vi "Configuracion_ADS_operar.vi"(7 "Direccion":i16, 9 "Configuracion ADS1263":T1 {"Muestras" items=["50", "250", "1000", "2000", "5000", "10000", "15000", "30000"]; "PGA" items=["1", "2", "4", "8", "16", "32"]; "Muestreo" items=["2.5 SPS", "5 SPS", "10 SPS", "16.6 SPS", "20 SPS", "50 SPS", "60 SPS", "100 SPS", "400 SPS", "1200 SPS", "2400 SPS", "4800 SPS", "7200 SPS", "14400 SPS", "19200 SPS", "38400 SPS"]}, 10 "ENVIAR_CONFI":bool) -> (1 "Muestras":i32, 2 "Configuracion":string)   [LabVIEW 2022 SP3]
panel:
  # "Velocidad de muestreo"
  # "PGA del sistema"
  # "HABILITAR MODO DIFERENCIAL 1 Y 2"
  # "HABILITAR MODO DIFERENCIAL 3 Y 4"
  # "FILTRO PARA AC1 Y AC2"
  # "100Hz"
  # "500Hz"
  # "FILTRO PARA AC3 Y AC4"
  # "100Hz"
  # "500Hz"
  # "MODO DE OPERACION DEMANDA"
  # "MODO DE OPERACION CONTROLADA"
  # "Cantidad de muestras tomadas"
  # "Recibir por LoRa"
  # "Recibir por SD"
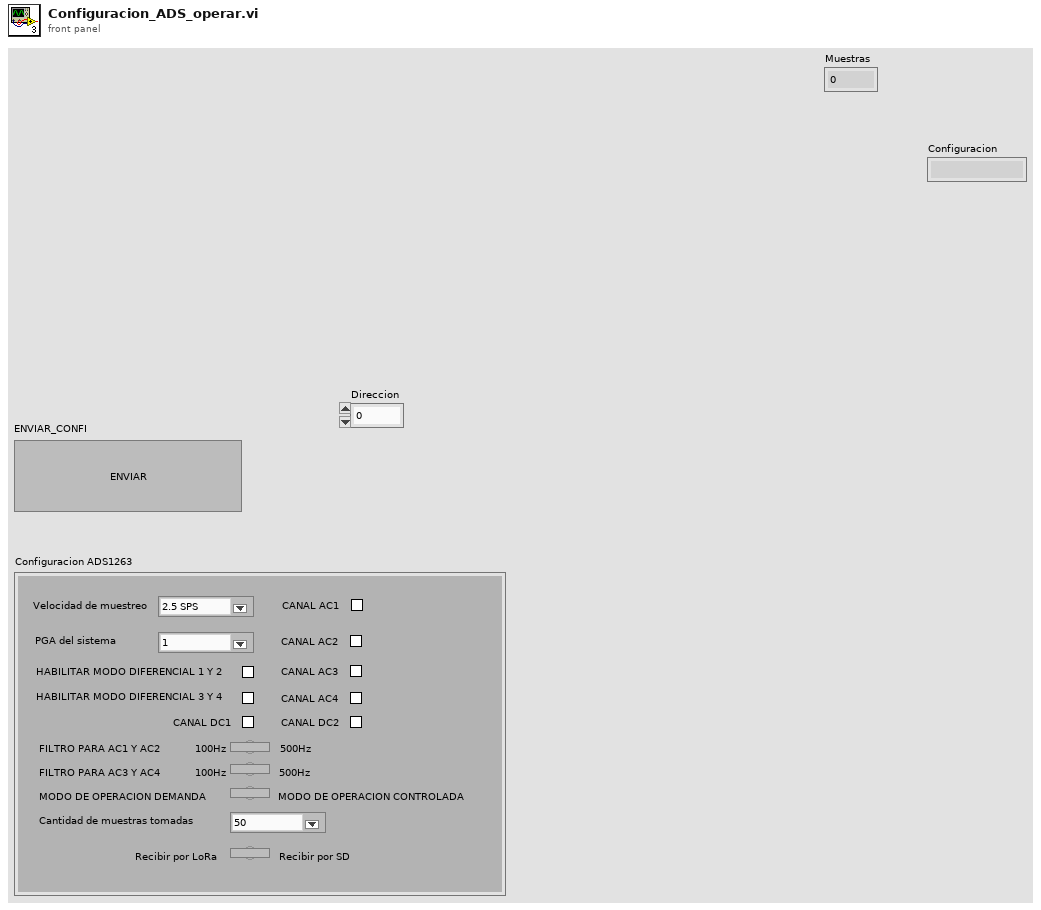
[diagram p1: front panel]
types:
  T1 = cluster{"Muestreo":u32, "PGA":u32, "DIF1Y2":bool, "DIF3Y4":bool, "CANAL AC1":bool, "CANAL AC2":bool, "CANAL AC3":bool, "CANAL AC4":bool, "CANAL DC1":bool, "CANAL DC2":bool, "FILTRO1":bool, "FILTRO2":bool, "MODO OPERACION":bool, "Muestras":u32, "MODO transmision":bool}
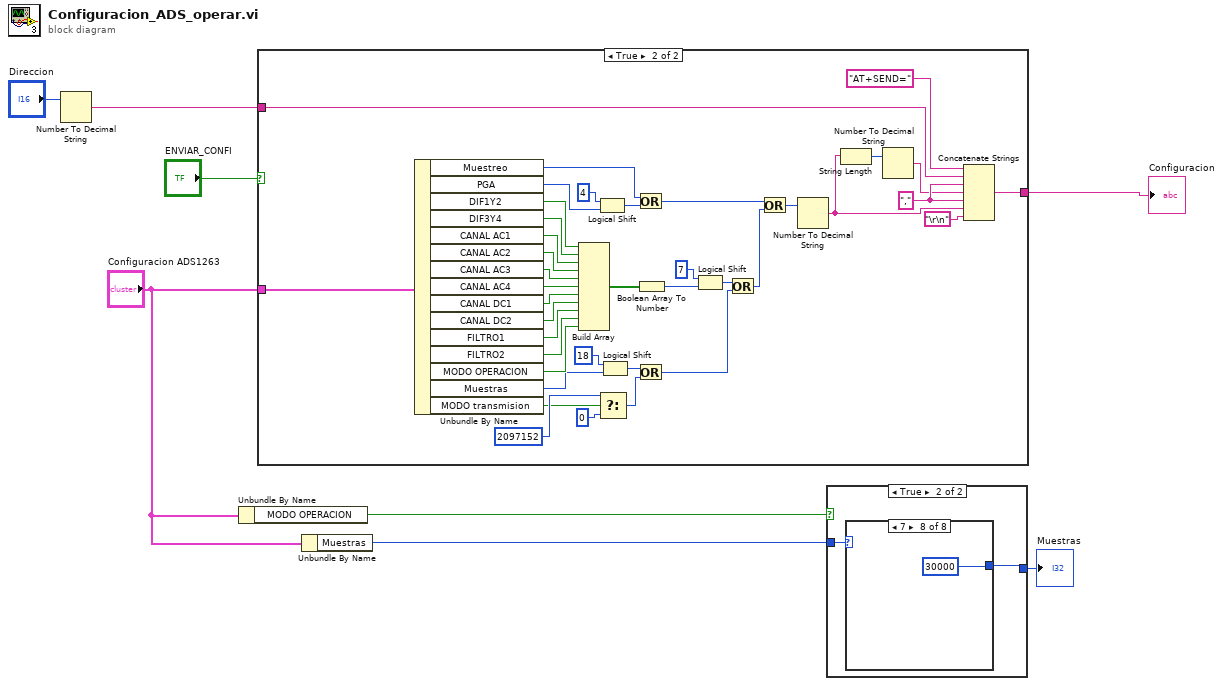
[diagram p0: block diagram]
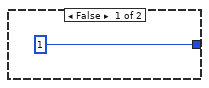
[diagram p2: hidden frame]
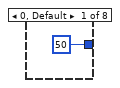
[diagram p3: hidden frame]
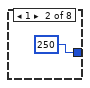
[diagram p4: hidden frame]
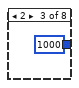
[diagram p5: hidden frame]
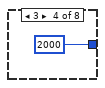
[diagram p6: hidden frame]
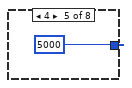
[diagram p7: hidden frame]
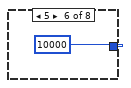
[diagram p8: hidden frame]
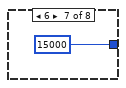
[diagram p9: hidden frame]
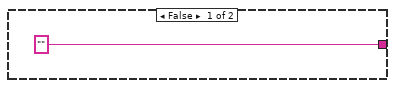
[diagram p10: hidden frame]
diagram:
  n1 = Number To Decimal String(number="Direccion") -> (decimal integer string=w3:string)  [unwired: 1 in]
  n2 = Unbundle By Name("Configuracion ADS1263") -> ("MODO OPERACION"=w2:bool)
  n3 = case shown="True" "ENVIAR_CONFI" {
    tunnel: ["" w12] -> w7
    tunnel: "Configuracion ADS1263" -> [_ w11]
    tunnel: w3 -> [_ w10]
    frame False {
    }
    frame True {
      w16 = "," ("string")
      n4 = Unbundle By Name(w11) -> ("Muestreo"=w22:u32, "PGA"=w23:u32, "DIF1Y2"=w48:bool, "DIF3Y4"=w47:bool, "CANAL AC1"=w46:bool, "CANAL AC2"=w45:bool, "CANAL AC3"=w44:bool, "CANAL AC4"=w43:bool, "CANAL DC1"=w42:bool, "CANAL DC2"=w41:bool, "FILTRO1"=w40:bool, "FILTRO2"=w39:bool, "MODO OPERACION"=w38:bool, "Muestras"=w33:u32, "MODO transmision"=w30:bool)
      n5 = Build Array(w48, w47, w46, w45, w44, w43, w42, w41, w40, w39, w38) -> (w35:bool[])
      n6 = Logical Shift(y=i16 4, x=w23) -> (x << y=w24:u32)
      n7 = Select(t=u32 2097152 ("y"), s=w30, f=u32 0 ("y")) -> (s? t:f=w28:u32)
      n8 = Logical Shift(y=i16 18, x=w33) -> (x << y=w29:u32)
      n9 = Or(x=w22, y=w24) -> (x .or. y?=w21:u32)
      n10 = Or(x=w29, y=w28) -> (x .or. y?=w26:u32)
      n11 = Boolean Array To Number(Boolean array=w35) -> (number=w36:u32)
      n12 = Logical Shift(y=i16 7, x=w36) -> (x << y=w27:u32)
      n13 = Or(x=w27, y=w26) -> (x .or. y?=w20:u32)
      n14 = Or(x=w21, y=w20) -> (x .or. y?=w19:u32)
      n15 = Number To Decimal String(number=w19) -> (decimal integer string=w13:string)  [unwired: 1 in]
      n16 = String Length(string=w13) -> (length=w18:i32)
      n17 = Number To Decimal String(number=w18) -> (decimal integer string=w15:string)  [unwired: 1 in]
      n18 = Concatenate Strings("AT+SEND=" ("string"), w10, w16, w15, w16, w13, "\r\n") -> (w12:string)
    }
  }
  "Configuracion" <- w7
  n19 = Unbundle By Name("Configuracion ADS1263") -> ("Muestras"=w5:u32)
  n20 = case shown="True" w2 {
    tunnel: w5 -> [_ w51]
    tunnel: [1 w50] -> w1
    frame False {
    }
    frame True {
      n21 = case shown="7" w51 {
        tunnel: [50 250 1000 2000 5000 10000 15000 30000] -> w50
        frame 0, Default {
        }
        frame 1 {
        }
        frame 2 {
        }
        frame 3 {
        }
        frame 4 {
        }
        frame 5 {
        }
        frame 6 {
        }
        frame 7 {
        }
      }
    }
  }
  "Muestras" <- w1
